vi "Measure Line Scan.vi"(7 "number of samples per channel":i32=-1, 8 "error in":errorcluster, 9 "Iterator":dbl, 10 "task/channels in":refnum<k21>, 11 "Array in":dbl[](array[numeric])) -> (0 "error out":errorcluster, 1 "mean":dbl format="%0.2f", 2 "task out":refnum<k21>, 3 "Array out":dbl[](array[numeric]))   [LabVIEW 2021]
uses:
  <vilib>/DAQmx/read.llb/DAQmx Read (Analog 1D DBL 1Chan NSamp).vi
  <vilib>/Analysis/baseanly.llb/Mean (DBL).vi
  <vilib>/DAQmx/miscellaneous.llb/DAQmx Fill In Error Info.vi
  <vilib>/Analysis/NI_AALBase.lvlib
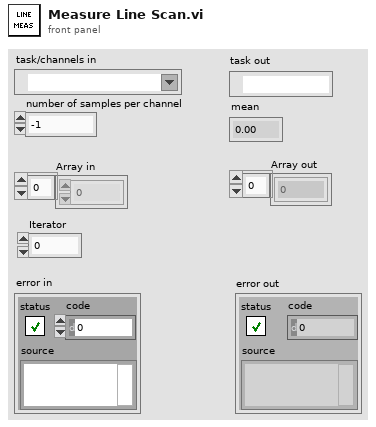
[diagram p1: front panel]
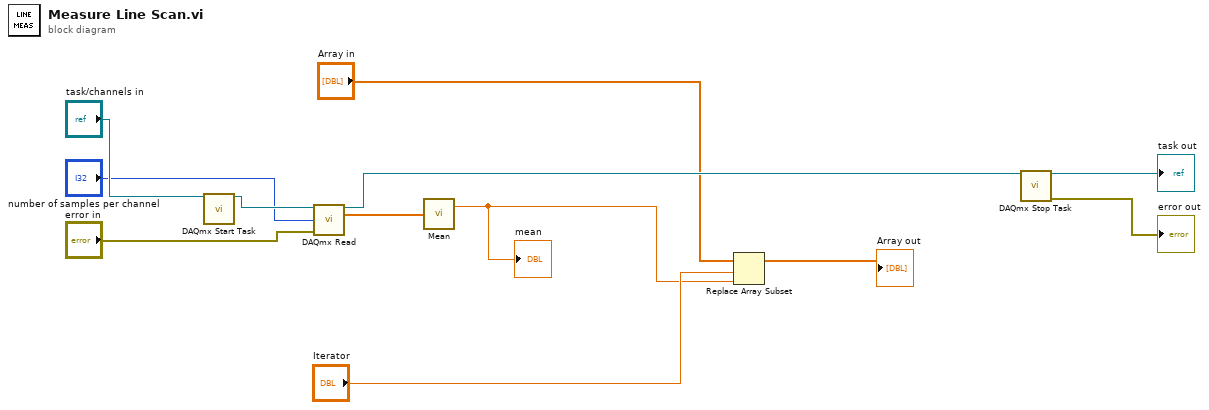
[diagram p0: block diagram]
diagram:
  n1 = call <vilib>:"DAQmx Start Task.vi"("task/channels in"="task/channels in") -> ("task out"=w11:refnum<k21>)  [unwired: 13 in, 1 out]
  n2 = call-poly <vilib>:"DAQmx Read.vi"("task/channels in"=w11, "number of samples per channel"="number of samples per channel", "error in"="error in") -> ("task out"=w8:refnum<k21>, "data"=w7:dbl[])  [unwired: 10 in, 1 out]
  n3 = call-poly <vilib>:"Mean.vi"("X"=w7) -> ("mean"=w2:dbl)  [unwired: 1 out]
  "mean" <- w2
  n4 = Replace Array Subset(array="Array in", new element=w2, index="Iterator") -> (→"Array out":dbl[])
  n5 = call <vilib>:"DAQmx Stop Task.vi"("task/channels in"=w8) -> ("task out"=→"task out":refnum<k21>, "error out"=→"error out":errorcluster)  [unwired: 13 in]
